vi "SetStringValue.vi"(1 "error in (no error)":errorcluster, 2 "String Value":string, 3 "Feature Name":string, 4 "IGxDevice":refnum<k24>) -> (0 "error out":errorcluster)   [LabVIEW 2013, in "GxLVlib.lvlib"]
uses:
  GxLVlib.lvlib
  F:/GxILibrary/Labview/trunk/private/dev/src/C#/x86/GxLVLib/dll/GxIAPINET.dll
  private/dev/src/C#/x86/GxLVLib/dll/GxIAPINET.dll
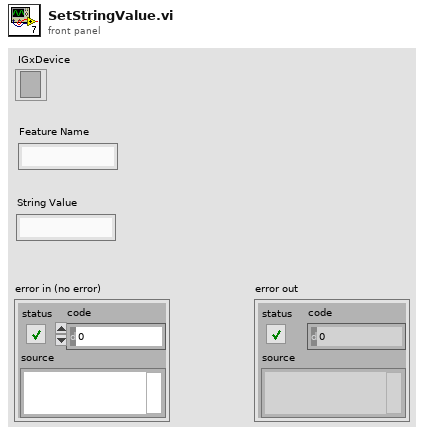
[diagram p1: front panel]
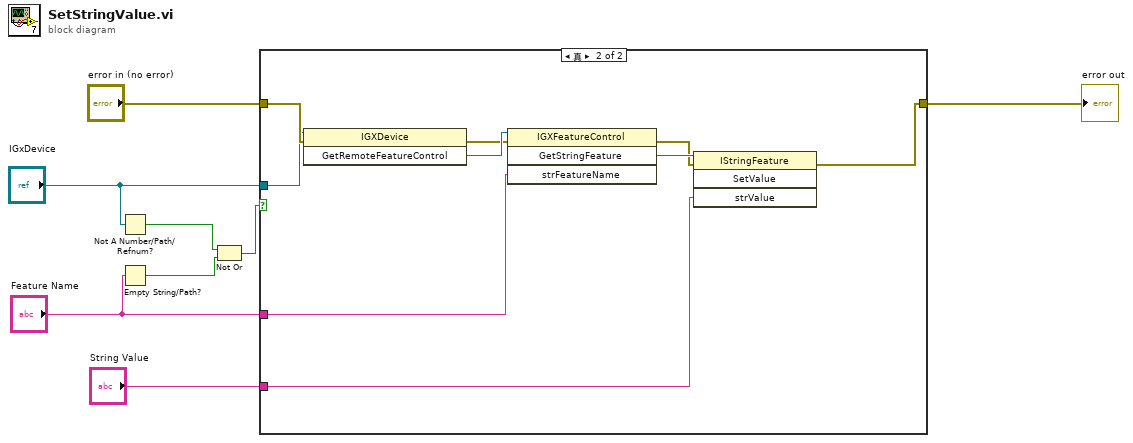
[diagram p0: block diagram]
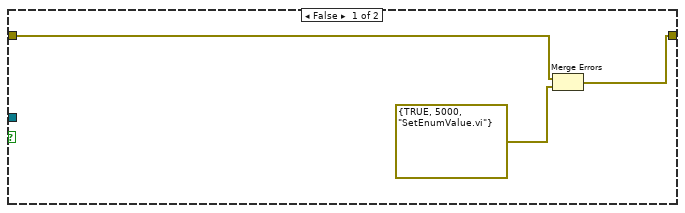
[diagram p2: hidden frame]
diagram:
  n1 = Not A Number/Path/Refnum?(number/path/refnum="IGxDevice") -> (NaN/Path/Refnum?=w8:bool)
  n2 = Empty String/Path?(string/path="Feature Name") -> (empty?=w7:bool)
  n3 = Not Or(1:w7, 2:w8) -> (0:w6:bool)
  n4 = case shown="真" w6 {
    tunnel: "error in (no error)" -> [w10 w20]
    tunnel: [w9 w12] -> w4
    tunnel: "IGxDevice" -> [_ w19]
    tunnel: "Feature Name" -> [_ w16]
    tunnel: "String Value" -> [_ w13]
    frame False {
      n5 = Merge Errors(w10, errorcluster {TRUE, 5000, "SetEnumValue.vi"}) -> (w9:errorcluster)
    }
    frame True {
      n6 = invoke class="IGXDevice" method="GetRemoteFeatureControl"(reference=w19, error in=w20) -> (error out=w17:errorcluster, "GetRemoteFeatureControl"=w18:refnum<k24>)  [unwired: 1 in, 1 out]
      n7 = invoke class="IGXFeatureControl" method="GetStringFeature"(reference=w18, error in=w17, "strFeatureName"=w16) -> (error out=w14:errorcluster, "GetStringFeature"=w15:refnum<k24>)  [unwired: 1 in, 2 out]
      n8 = invoke class="IStringFeature" method="SetValue"(reference=w15, error in=w14, "strValue"=w13) -> (error out=w12:errorcluster)  [unwired: 1 in, 3 out]
    }
  }
  "error out" <- w4
